vi "Util_GetTime_U64.vi"(8 "error in (no error)":void) -> (0 "error out":T2, 3 "FPGA_Time_MicroSeconds":numeric format="%.0g")   [LabVIEW 2019, in "Trajectory_Library.lvlib"]
doc: "This subVI returns both words of the FPGA continuously running elapsed time in microseconds.\n\nThis is an internal routine and should NOT be called directly by the end user. \n\nOn the RoboRIO this reads the high resolution FPGA time. The resolution, not accuracy, of the FPGA timer is 1 microsecond. The normal FPGA clock register (32 bits) rolls over approximately every 71 minutes. To significantly extend the rollover time,, this routine reads both the high and low FPGA clock registers. High/low register turnover read sequencing is dealt with by reading the high register twice, once before and once after the low register. If the values are different, the read is repeated to assure consistency between the high and low values. On a PC the standard operating system timer with 1 millisecond resolution is used. \n\nNOTES:\n--------\n- Set a conditional complilation variable TRAJLIB_USEOSTIME and set it to a value of 1 to force this routine to read the RoboRIO operating system time instead of the FPGA time. This will have 1 millisecond resolution. This routine executes faster, approx 1 microsecond.\n\n - On the RoboRIO there is some drift between the FPGA and operating system clocks. The drift isn't consistent, but appears to be approximately 20 milliseconds / hour. This isn't enough to be of concern.\n\n\nInput parameters:\n - Error In -- Error Data Cluster -- \n\nReturns:\n - FPGA_Time_Microseconds -- UInt64 -- Full 64 bit value of the continously counting FPGA clock.\n - Output Error -- Output error cluster. An error will be returned if there are problems reading the FPGA or of the FPGA clock high register changes twice while reading the value.\n\nCustom Errors:\n - 8020 -- The upper FPGA time register changed during both attempts to read the FPGA time values. The returned time may not be valid."
uses:
  Trajectory_Library.lvlib
  <vilib>/Rock Robotics/SystemInterfaces/System/FPGA_SystemFRC FPGA Ref.ctl
  <vilib>/rvi/interface/nirviReadWriteControl/nirviReadWriteControl.xnode
  NiFpgaLv.dll
  <vilib>/Utility/error.llb/Error Cluster From Error Code.vi
  <vilib>/rvi/interface/Simulation/niFpgaSimulationCallBeginRW.vi
  <vilib>/rvi/errors/niLvFpgaAdjustHostInterfaceError.vi
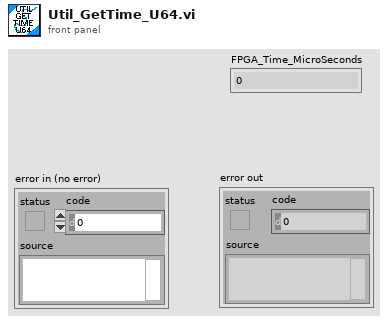
[diagram p1: front panel]
types:
  T1 = typedef "niFpgaNodeNameForErrorReporting.ctl" = enum16{"Open FPGA VI Reference", "Read/Write Control", "Invoke Method: Abort", "Invoke Method: Acknowledge IRQ", "Invoke Method: Download", "Invoke Method: FIFO.Configure", "Invoke Method: FIFO.Read", "Invoke Method: FIFO.Start", "Invoke Method: FIFO.Stop", "Invoke Method: FIFO.Write", "Invoke Method: Reset", "Invoke Method: Run", "Invoke Method: Wait on IRQ", "Close FPGA VI Reference", "Invoke Method: FIFO.Acquire Read Region", "Invoke Method: FIFO.Acquire Write Region"}
  T2 = cluster{"source":string, "code":numeric, "status":boolean}
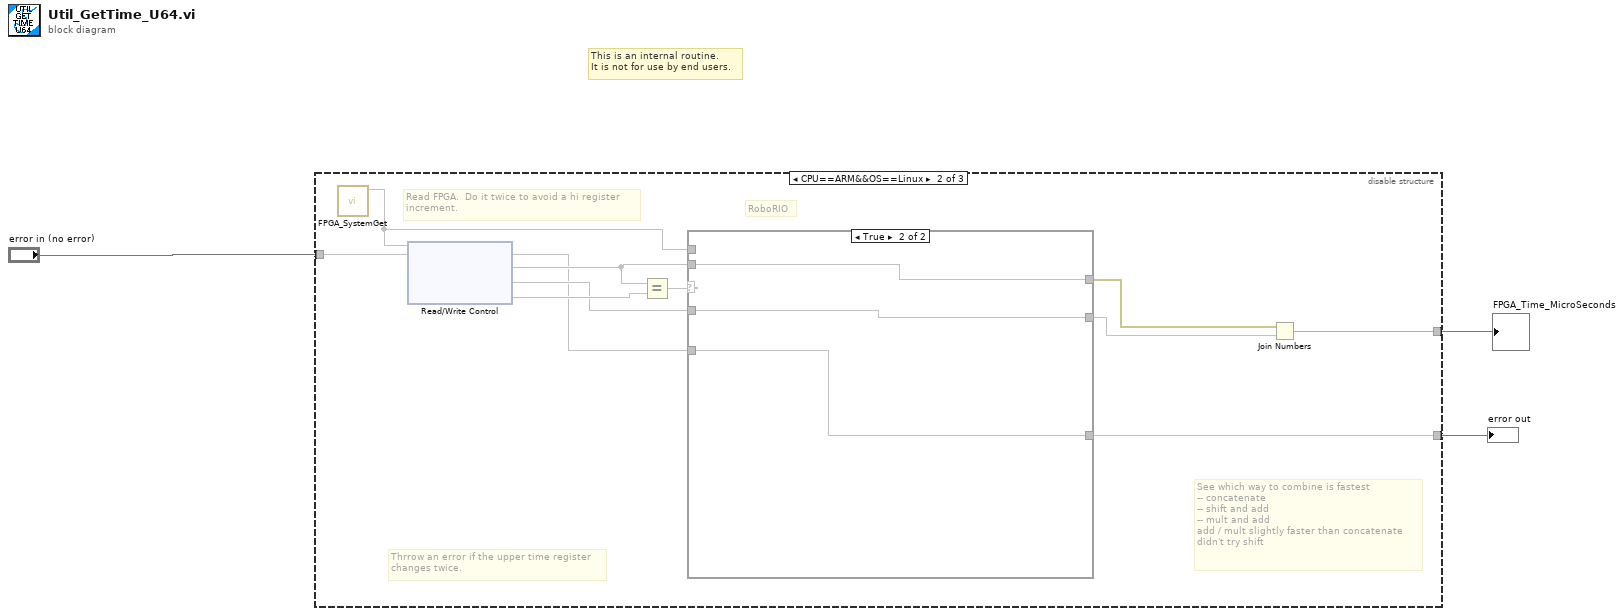
[diagram p0: block diagram]
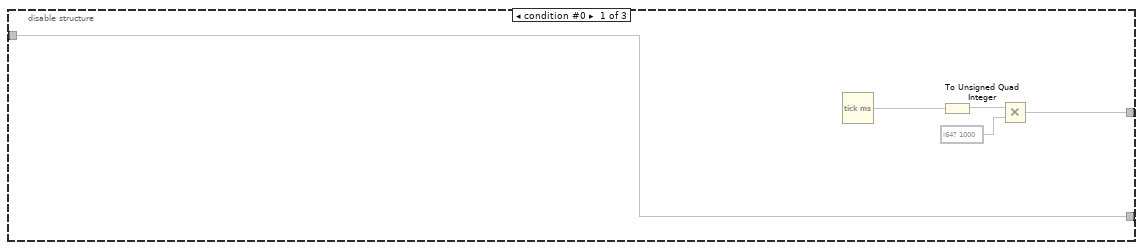
[diagram p2: hidden frame]
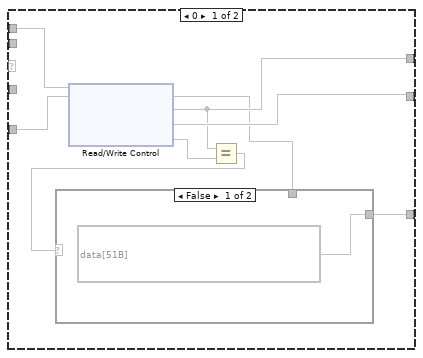
[diagram p3: hidden frame]
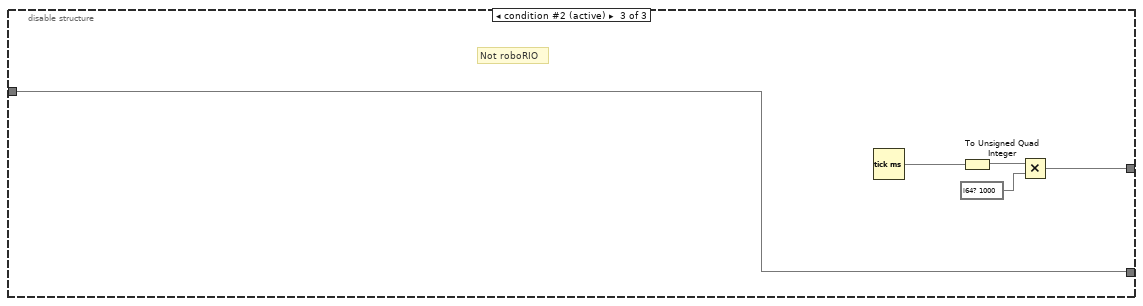
[diagram p5: hidden frame]
diagram:
  # "This is an internal routine.   \nIt is not for use by end users."
  n1 = disable-structure shown="CPU==ARM&&OS==Linux" {
    disable-tunnel: "error in (no error)" -> [w8 w12 w37]
    disable-tunnel: [w8 w15 w37] -> w2
    disable-tunnel: [w4 w9 w33] -> w1
    frame condition #0 {
      n2 = Tick Count (ms)() -> (millisecond timer value=w7)
      n3 = To Unsigned Quad Integer(1:w7) -> (0:w6)
      n4 = Multiply(x=w6, y=i64? 1000) -> (x*y=w4)
    }
    frame condition #1 {
      # "See which way to combine is fastest\n-- concatenate\n-- shift and add\n-- mult and add\nadd / mult slightly faster than concatenate\ndidn't try shift"
      # "RoboRIO"
      # "Read FPGA.  Do it twice to avoid a hi register\nincrement."
      # "Thrrow an error if the upper time register\nchanges twice."
      n5 = call <vilib>:"FPGA_SystemGet.vi"() -> (3:w13)  [unwired: 11 in]
      n6 = xnode "Read/Write Control"(w13, w12) -> (w14, w17, w16, w19)  [unwired: 1 out]
      n7 = Equal?(x=w17, y=w19) -> (x = y?=w18)
      n8 = case shown="True" w18 {
        tunnel: [w24 w32] -> w11
        tunnel: w17 -> [_ w32]
        tunnel: [w25 w31] -> w10
        tunnel: w16 -> [_ w31]
        tunnel: [w21 w30] -> w15
        tunnel: w14 -> [w26 w30]
        tunnel: w13 -> [w27 _]
        frame 0 {
          n9 = xnode "Read/Write Control"(w27, w26) -> (w20, w24, w25, w23)  [unwired: 1 out]
          n10 = Equal?(x=w24, y=w23) -> (x = y?=w22)
          n11 = case shown="False" w22 {
            tunnel: [data[51B] ("error out") w29] -> w21
            tunnel: w20 -> [_ w29]
            frame 0 {
            }
            frame 1 {
            }
          }
        }
        frame 1 {
        }
      }
      n12 = Join Numbers(hi=w11, lo=w10) -> ((hi.lo)=w9:T1)
    }
    frame condition #2 (active) {
      # "Not roboRIO"
      n13 = Tick Count (ms)() -> (millisecond timer value=w34)
      n14 = To Unsigned Quad Integer(1:w34) -> (0:w36)
      n15 = Multiply(x=w36, y=i64? 1000) -> (x*y=w33)
    }
  }
  "error out" <- w2
  "FPGA_Time_MicroSeconds" <- w1
